vi "isAngleBetween.vi"(9 "End":dbl, 10 "Start":dbl, 11 "Angle":dbl(knob) scale=180.0..-180.0) -> (2 "Clockwise?":bool, 3 "Between?":bool)   [LabVIEW 2017]
panel:
  out "x-y":dbl
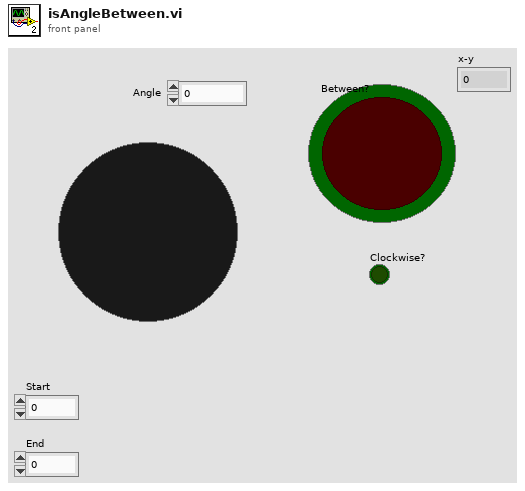
[diagram p1: front panel]
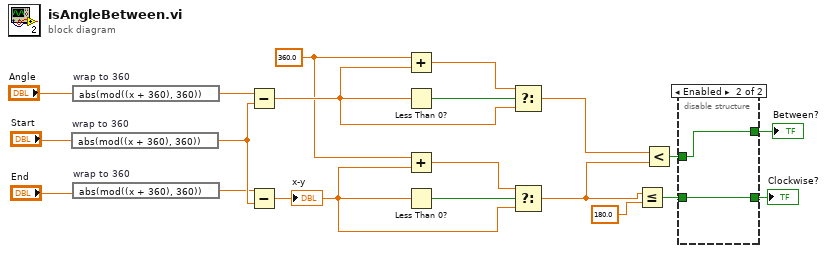
[diagram p0: block diagram]
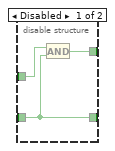
[diagram p2: hidden frame]
diagram:
  w17 = 360.0
  n1 = expression code="abs(mod((x + 360), 360))" "wrap to 360"("Start") -> (w4:dbl)
  n2 = expression code="abs(mod((x + 360), 360))" "wrap to 360"("Angle") -> (w6:dbl)
  n3 = expression code="abs(mod((x + 360), 360))" "wrap to 360"("End") -> (w2:dbl)
  n4 = Subtract(x=w6, y=w4) -> (x-y=w18:dbl)
  n5 = Subtract(x=w2, y=w4) -> (x-y=w16:dbl)
  "x-y" <- w16
  n6 = Add(x=w17, y=w18) -> (x+y=w15:dbl)
  n7 = Less Than 0?(x=w18) -> (x < 0?=w14:bool)
  n8 = Add(x=w17, y=w16) -> (x+y=w19:dbl)
  n9 = Less Than 0?(x=w16) -> (x < 0?=w13:bool)
  n10 = Select(t=w15, s=w14, f=w18) -> (s? t:f=w9:dbl)
  n11 = Select(t=w19, s=w13, f=w16) -> (s? t:f=w8:dbl)
  n12 = Less Or Equal?(x=w8, y=180.0) -> (x <= y?=w10:bool)
  n13 = Less?(x=w9, y=w8) -> (x < y?=w20:bool)
  n14 = disable-structure shown="Enabled" {
    disable-tunnel: w20 -> [w23 w25]
    disable-tunnel: [w22 w25] -> w11
    disable-tunnel: w10 -> [w21 w24]
    disable-tunnel: [w21 w24] -> w1
    frame Disabled {
      n15 = And(x=w23, y=w21) -> (x .and. y?=w22:bool)
    }
    frame Enabled {
    }
  }
  "Between?" <- w11
  "Clockwise?" <- w1
